vi "GhettoClimb.vi"(8 "error in (no error)":errorcluster, 11 "Elevator Concrete in":refnum<class "Elevator Arm.lvclass">) -> (0 "error out":errorcluster, 3 "Elevator Concrete out":refnum<class "Elevator Arm.lvclass">)   [LabVIEW 2018, in "Elevator.lvlib" / "Elevator Arm.lvclass"]
uses:
  Elevator Arm.lvclass
  C:/Users/Public/Documents/2019DeepSpace/Classes/Elevator/Elevator.lvclass
  <vilib>/Rock Robotics/WPI/ThirdParty/Phoenix-LabVIEW/Motor Controller/Controls/CTRE_Phoenix_MotorControl_ControlMode.ctl
  Elevator Arm.lvclass/Elevator Arm.ctl
  Elevator.lvclass
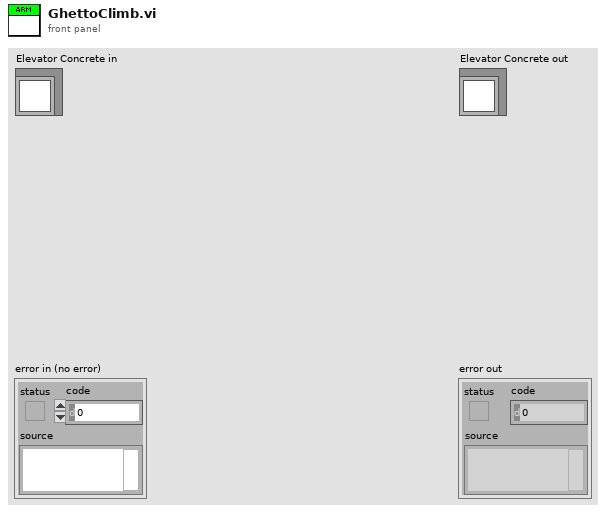
[diagram p1: front panel]
types:
  T1 = typedef "CTRE_Phoenix_MotorControl_ControlMode.ctl" = u16
  T2 = typedef "Elevator.lvlib/Elevator.lvclass/Elevator Constants.ctl" = cluster{"Arm Motion Magic Max Velocity":u32, "Arm Motion Magic Max Acceleration":u32, "Wrist Motion Magic Max Velocity":u32, "Wrist Motion Magic Max Acceleration":u32, "Elevator Linear Motion Magic Max Velocity":u32, "Elevator Linear Motion Magic Max Acceleration":u32, "Arm Gear Ratio":dbl, "Wrist Gear Ratio":dbl, "Elevator Linear Gear Ratio":dbl, "Arm Encoder ABS Value":i32, "Wrist Encoder ABS Value":i32}
  T3 = typedef "WPI_MotorControlDeviceRef.ctl" = cluster{"DeviceStatus":errorcluster, "Type":T4, "PWM":cluster{"PWM Channel":T5, "DeadBand":T6}, "CAN":cluster{"Device Number":u8, "SetOutput VI Ref":variant, "GetOutput VI Ref":variant, "Enable VI Ref":variant, "Disable VI Ref":variant, "Data":variant}, "Invert":bool, "DIO PWM":cluster{"PWM \"Enable\" Channel":T5, "DIOChannel":T7, "PWM Rate":dbl}}
  T4 = typedef "WPI_MotorControlType.ctl" = enum16{"PWM", "CAN", "DIO PWM"}
  T5 = typedef "FPGA_DIOPWMChannel.ctl" = enum8{"PWM 0", "PWM 1", "PWM 2", "PWM 3", "PWM 4", "PWM 5", "PWM 6", "PWM 7", "PWM 8", "PWM 9", "PWM MXP 0", "PWM MXP 1", "PWM MXP 2", "PWM MXP 3", "PWM MXP 4", "PWM MXP 5", "PWM MXP 6", "PWM MXP 7", "PWM MXP 8", "PWM MXP 9", "Invalid"}
  T6 = typedef "WPI_PWMDeadband.ctl" = cluster{"Name":string, "maxPositivePwm":i32, "minPositivePwm":i32, "centerPwm":i32, "maxNegativePwm":i32, "minNegativePwm":i32, "angularRange":u16}
  T7 = typedef "FPGA_DIOChannel.ctl" = enum8{"DIO 0", "DIO 1", "DIO 2", "DIO 3", "DIO 4", "DIO 5", "DIO 6", "DIO 7", "DIO 8", "DIO 9", "DIO MXP 0", "DIO MXP 1", "DIO MXP 2", "DIO MXP 3", "DIO MXP 4", "DIO MXP 5", "DIO MXP 6", "DIO MXP 7", "DIO MXP 8", "DIO MXP 9", "DIO MXP 10", "DIO MXP 11", "DIO MXP 12", "DIO MXP 13", "DIO MXP 14", "DIO MXP 15", "SPI Port CS1", "SPI Port CS2", "SPI Port CS3", "SPI Port MISO", "SPI Port MOSI", "Invalid"}
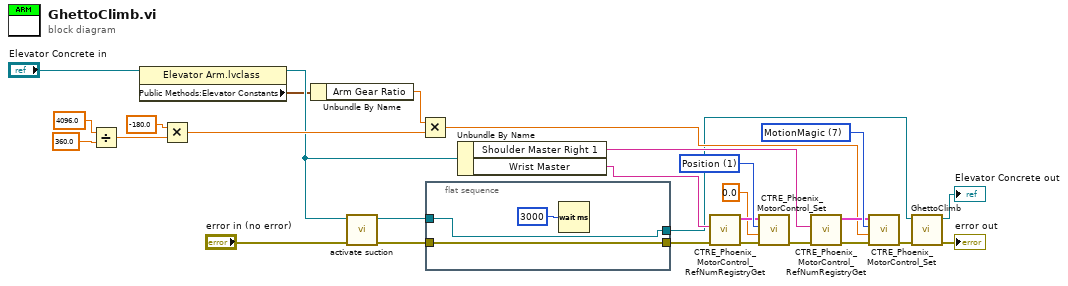
[diagram p0: block diagram]
diagram:
  w23 = T1 1 items=["PercentOutput"=0, "Position"=1, "Velocity"=2, "Current"=3, "Follower"=5, "MotionProfile"=6, "MotionMagic"=7, "MotionProfileArc"=10, "Disabled"=15] ("Control Mode")
  w26 = T1 7 items=["PercentOutput"=0, "Position"=1, "Velocity"=2, "Current"=3, "Follower"=5, "MotionProfile"=6, "MotionMagic"=7, "MotionProfileArc"=10, "Disabled"=15] ("Control Mode")
  n1 = Divide(x=4096.0, y=360.0) -> (x/y=w17:dbl)
  n2 = property class="Elevator Arm.lvclass"(reference="Elevator Concrete in") -> (reference out=w3:refnum<class "Elevator Arm.lvclass">, "Public Methods:Elevator Constants"=w2:T2)  [unwired: 1 in, 1 out]
  n3 = Multiply(x=-180.0, y=w17) -> (x*y=w16:dbl)
  n4 = Unbundle By Name(w2) -> ("Arm Gear Ratio"=w1:dbl)
  n5 = call "activate suction.vi"("error in (no error)"="error in (no error)", "Elevator Concrete in"=w3) -> ("error out"=w4:errorcluster, "Elevator Concrete out"=w6:refnum<class "Elevator Arm.lvclass">)  [unwired: 8 in]
  n6 = Multiply(x=w1, y=w16) -> (x*y=w15:dbl)
  n7 = flat-sequence {
    tunnel: [w31] -> w7
    tunnel: w6 -> [w31]
    tunnel: [w30] -> w5
    tunnel: w4 -> [w30]
    frame #0 {
      n8 = Wait (ms)(milliseconds to wait=u32 3000) -> ()  [unwired: 1 out]
    }
  }
  n9 = Unbundle By Name(w3) -> ("Shoulder Master Right 1"=w12:string, "Wrist Master"=w11:string)
  n10 = call <vilib>:"CTRE_Phoenix_MotorControl_RefNumRegistryGet.vi"("error in (no error)"=w5, "refnum name"=w11) -> ("error out"=w21:errorcluster, "PhoenixMotorControlDevRef"=w22:T3)  [unwired: 8 in]
  n11 = call <vilib>:"CTRE_Phoenix_MotorControl_Set.vi"("error in (no error)"=w21, "Output"=0.0, "Control Mode"=w23, "PhoenixMotorControlDevRef"=w22) -> ("error out"=w13:errorcluster)  [unwired: 6 in, 1 out]
  n12 = call <vilib>:"CTRE_Phoenix_MotorControl_RefNumRegistryGet.vi"("error in (no error)"=w13, "refnum name"=w12) -> ("error out"=w24:errorcluster, "PhoenixMotorControlDevRef"=w25:T3)  [unwired: 8 in]
  n13 = call <vilib>:"CTRE_Phoenix_MotorControl_Set.vi"("error in (no error)"=w24, "Output"=w15, "Control Mode"=w26, "PhoenixMotorControlDevRef"=w25) -> ("error out"=w9:errorcluster)  [unwired: 6 in, 1 out]
  n14 = call-parent "GhettoClimb.vi"("error in (no error)"=w9, "Elevator in"=w7) -> ("error out"=→"error out":errorcluster, "Elevator out"=→"Elevator Concrete out":refnum<class "Elevator Arm.lvclass">)  [unwired: 8 in]
